vi "simple_load_hdf5_map.vi"(8 "error in (no error)":errorcluster, 10 "Path":path, 11 "IntensityGraph in":refnum<vi>) -> (0 "error out":errorcluster)   [LabVIEW 2015, in "front_panel.lvclass"]
uses:
  front_panel.lvclass
  <vilib>/UPVI/lvhdf5/file.llb/LVH5F Operation.ctl
  rdbu_256.ctl
  <vilib>/Utility/miscctls.llb/LVRectTypeDef.ctl
  <vilib>/UPVI/lvhdf5/group.llb/H5G_obj_t.ctl
  <vilib>/UPVI/lvhdf5/dataset.llb/LVH5D Operation.ctl
  <vilib>/UPVI/lvhdf5/utility.llb/Select HDF5 Dialog.vi
  <vilib>/UPVI/lvhdf5/utility.llb/Select HDF5 Dialog (Object Only).vi
  <vilib>/UPVI/lvhdf5/dataset.llb/Simple H5Dread (Variant).vi
  <vilib>/UPVI/lvhdf5/dataset.llb/Simple H5Dread.xnode
  <vilib>/UPVI/lvhdf5/library.llb/HDF5 Ref.ctl
  <vilib>/UPVI/lvhdf5/file.llb/H5Fopen.vi
  <vilib>/UPVI/lvhdf5/utility.llb/Select HDF5 Dialog (File and Object).vi
  <vilib>/UPVI/lvhdf5/identifier.llb/Not an HDF5 Refnum Constant.vi
  <vilib>/UPVI/lvhdf5/dataset.llb/OpenCreateReplace Dataset.vi
  <vilib>/UPVI/lvhdf5/dataset.llb/H5Dget_space.vi
  <vilib>/UPVI/lvhdf5/dataspace.llb/H5Sget_simple_extent_dims.vi
  <vilib>/UPVI/lvhdf5/dataspace.llb/H5Sselect_hyperslab.vi
  <vilib>/UPVI/lvhdf5/dataset.llb/H5Dread (Variant).vi
  <vilib>/UPVI/lvhdf5/attribute.llb/private/LVH5AreadWDTAttrs.vi
  <vilib>/UPVI/lvhdf5/dataspace.llb/H5Sclose.vi
  <vilib>/Utility/error.llb/Error Cluster From Error Code.vi
  <vilib>/UPVI/lvhdf5/dataset.llb/H5Dclose.vi
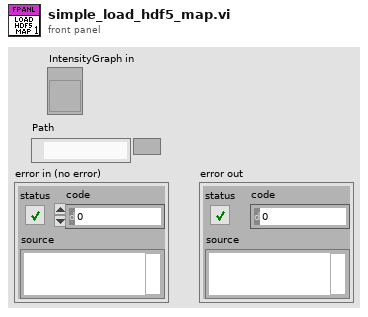
[diagram p1: front panel]
types:
  T1 = typedef "LVH5F Operation.ctl" = enum16{"open", "open or create", "create or replace", "create or replace (with confirmation)", "create", "open (read only)"}
  T2 = typedef "LVRectTypeDef.ctl" = cluster{"Left":i16, "Top":i16, "Right":i16, "Bottom":i16}
  T3 = cluster{"Behavior":enum32{"Invalid", "Default", "Floating", "Floating/Auto-Hide", "Modal"}, "Position":T2, "Center":bool, "Title":string}
  T4 = typedef "LVH5D Operation.ctl" = enum16{"open", "replace", "create", "open or create", "create or replace", "create or replace with confirmation"}
  T5 = typedef "H5G_obj_t.ctl" = i32
  T6 = cluster{"Object Types (any)":T5[], "Object Pattern":string}
  T7 = typedef "rdbu_256.ctl" = u32[]
  T8 = typedef "HDF5 Ref.ctl" = refnum<k1>
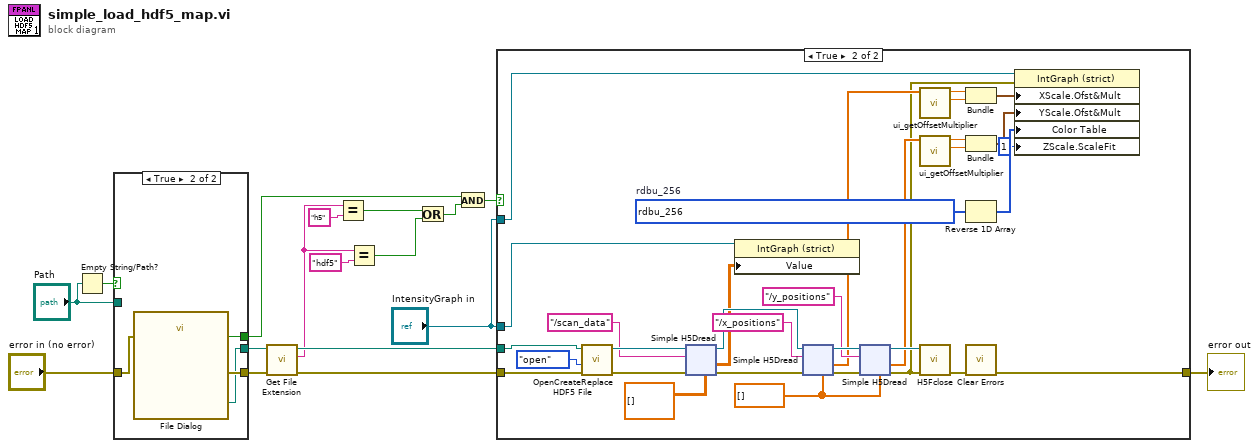
[diagram p0: block diagram]
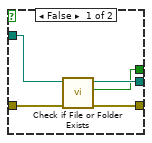
[diagram p2: hidden frame]
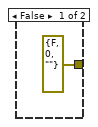
[diagram p3: hidden frame]
diagram:
  n1 = Empty String/Path?(string/path="Path") -> (empty?=w2:bool)
  n2 = case shown="True" w2 {
    tunnel: [w19 w26] -> w13
    tunnel: [w20 w25] -> w6
    tunnel: [w21 w24] -> w5
    tunnel: "error in (no error)" -> [w18 w23]
    tunnel: "Path" -> [w22 _]
    frame False {
      n3 = call <vilib>:"Check if File or Folder Exists.vi"("error in (no error)"=w18, "path"=w22) -> ("error out"=w20:errorcluster, "file or folder exists?"=w19:bool, "dup path"=w21:path)  [unwired: 7 in]
    }
    frame True {
      n4 = call "File Dialog"("error in"=w23) -> ("selected path"=w24:path, "exists"=w26:bool, "error out"=w25:errorcluster)  [unwired: 11 in, 1 out]
    }
  }
  n5 = call <vilib>:"Get File Extension.vi"("error in (no error)"=w6, "file"=w5) -> ("error out"=w15:errorcluster, "lowercase file extension"=w8:string, "dup file"=w16:path)  [unwired: 5 in, 2 out]
  n6 = Equal?(x=w8, y="h5") -> (x = y?=w11:bool)
  n7 = Equal?(x=w8, y="hdf5") -> (x = y?=w10:bool)
  n8 = Or(x=w11, y=w10) -> (x .or. y?=w14:bool)
  n9 = And(x=w13, y=w14) -> (x .and. y?=w12:bool)
  n10 = case shown="True" w12 {
    tunnel: w15 -> [_ w58]
    tunnel: w16 -> [_ w57]
    tunnel: [errorcluster {"status"=FALSE, "code"=0, "source"=""} ("error out") w46] -> w17
    tunnel: "IntensityGraph in" -> [_ w30]
    tunnel: "IntensityGraph in" -> [_ w29]
    frame False {
    }
    frame True {
      w32 = T7 [6750239, 6947103, 7143968, 7340832, 7537697, 7734561, 7931426, 8128290, 8325155, 8522019, 8718884, 8915748, 9112613, 9309221, 9506086, 9702950, 9899815, 10096679, 10293544, 10490408, 10687273, 10884137, 11081002, 11277866, 11474731, 11671595, 11671595, 11737900, 11869742, 11936047, 12067888, 12133938, 12265779, 12332085, 12463926, 12530231, 12596537, 12728378, 12794683, 12926269, 12992574, 13124415, 13190721, 13257026, 13388867, 13455173, 13587014, 13653064, 13784905, 13851210, 13983052, 14049357, 14049357, 14115663, 14181969, 14313555, 14379861, 14446168, 14512474, 14578524, 14710366, 14776672, 14842978, 14909028, 14975334, 15107177, 15173483, 15239533, 15305839, 15372145, 15503987, 15570037, 15636343, 15702650, 15768956, 15900542, 15966848, 16033154, 16033154, 16033669, 16099720, 16100234, 16101005, 16167056, 16167571, 16233621, 16234136, 16234651, 16300958, 16301472, 16301987, 16368038, 16368553, 16369067, 16435374, 16435889, 16436404, 16502454, 16502969, 16569020, 16569791, 16570305, 16636356, 16636871, 16636871, 16637129, 16637387, 16572109, 16572367, 16572881, 16573139, 16507860, 16508118, 16508376, 16508634, 16443356, 16443614, 16444128, 16444386, 16379108, 16379366, 16379624, 16379882, 16314603, 16314861, 16315375, 16315633, 16250355, 16250613, 16250871, 16250871, 16119543, 16054006, 15922678, 15856886, 15725558, 15660021, 15528693, 15462901, 15331828, 15266036, 15134708, 15068916, 14937843, 14872051, 14740723, 14674931, 14543858, 14478066, 14346738, 14281201, 14149873, 14084081, 13952753, 13887216, 13755888, 13755888, 13559023, 13427438, 13230574, 13033709, 12902124, 12705260, 12573931, 12376810, 12179945, 12048616, 11851496, 11720167, 11523302, 11326182, 11194853, 10997988, 10800867, 10669538, 10472674, 10275553, 10144224, 9947360, 9815775, 9618910, 9618910, 9421789, 9159132, 8962011, 8764890, 8567768, 8304855, 8107734, 7910613, 7647956, 7450835, 7253714, 6991056, 6793935, 6596814, 6399693, 6137036, 5939915, 5742794, 5479881, 5282760, 5085638, 4888517, 4625860, 4428739, 4428739, 4362690, 4231105, 4165056, 4033727, 3967678, 3836093, 3770044, 3703995, 3572410, 3506361, 3374776, 3308728, 3242935, 3111350, 3045301, 2913716, 2847667, 2781618, 2650033, 2584240, 2452655, 2386606, 2255021, 2188972, 2188972, 2122921, 2056870, 1990563, 1858976, 1792924, 1726617, 1660566, 1594515, 1462928, 1396877, 1330570, 1264518, 1198467, 1132160, 1066109, 934522, 868471, 802420, 736113, 670062, 538474, 472167, 406116, 340065]  # rdbu_256
      w43 = dbl[] []
      n11 = call <vilib>:"OpenCreateReplace HDF5 File.vi"("error in (no error)"=w58, "function (open or create)"=LVH5F_Operation."open", "path"=w57) -> ("error out"=w55:errorcluster, "HDF5 Ref out"=w56:T8)  [unwired: 5 in]
      n12 = xnode "Simple H5Dread"("Dataset Path"="/scan_data", "error in (no error)"=w55, "HDF5 Path or Ref"=w56, "Data"=dbl[][] []) -> ("HDF5 Ref out"=w52:T8, "error out"=w51:errorcluster, "Data out"=w42:dbl[][])  [unwired: 1 out]
      n13 = property class="IntGraph (strict)"(reference=w30, "Value"=w42) -> ()  [unwired: 1 in, 2 out]
      n14 = xnode "Simple H5Dread"("Dataset Path"="/x_positions", "error in (no error)"=w51, "HDF5 Path or Ref"=w52, "Data"=w43) -> ("HDF5 Ref out"=w49:T8, "error out"=w50:errorcluster, "Data out"=w40:dbl[])  [unwired: 1 out]
      n15 = xnode "Simple H5Dread"("Dataset Path"="/y_positions", "error in (no error)"=w50, "HDF5 Path or Ref"=w49, "Data"=w43) -> ("HDF5 Ref out"=w48:T8, "error out"=w35:errorcluster, "Data out"=w41:dbl[])  [unwired: 1 out]
      n16 = call "ui_getOffsetMultiplier.vi"("Axis"=w40) -> ("Multiplier"=w36:dbl, "Offset"=w37:dbl)  [unwired: 9 in]
      n17 = call "ui_getOffsetMultiplier.vi"("Axis"=w41) -> ("Multiplier"=w38:dbl, "Offset"=w39:dbl)  [unwired: 9 in]
      n18 = call <vilib>:"H5Fclose.vi"("error in (no error)"=w35, "HDF5 Ref"=w48) -> ("error out"=w47:errorcluster)  [unwired: 7 in]
      n19 = Bundle("Offset"=w37, "Multiplier"=w36) -> (w33:cluster{"Offset":dbl, "Multiplier":dbl})  [unwired: 1 in]
      n20 = Bundle("Offset"=w39, "Multiplier"=w38) -> (w34:cluster{"Offset":dbl, "Multiplier":dbl})  [unwired: 1 in]
      n21 = Reverse 1D Array(array=w32) -> (reversed array=w31:T7)
      n22 = call <vilib>:"Clear Errors.vi"("error in (no error)"=w47) -> ("error out"=w46:errorcluster)  [unwired: 5 in, 1 out]
      n23 = property on="Property Node" class="IntGraph (strict)"(reference=w29, error in=w35, "XScale.Ofst&Mult"=w33, "YScale.Ofst&Mult"=w34, "Color Table"=w31, "ZScale.ScaleFit"=u8 1 ("Z Scale.Scale Fit")) -> ()  [unwired: 2 out]
    }
  }
  "error out" <- w17
